vi "voltageScan.vi"(8 "error in (no error)":errorcluster, 11 "VISA Refnum in":refnum<visa-resource-name>) -> (0 "error out":errorcluster, 2 "stringVoltage":string, 3 "numberVoltage":dbl)   [LabVIEW 2018]
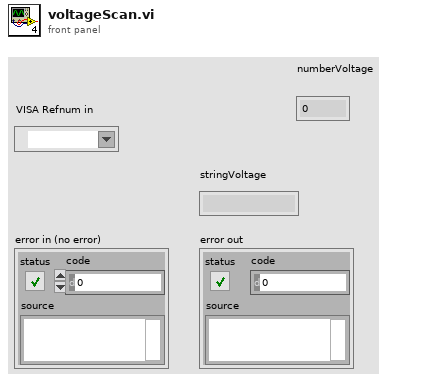
[diagram p1: front panel]
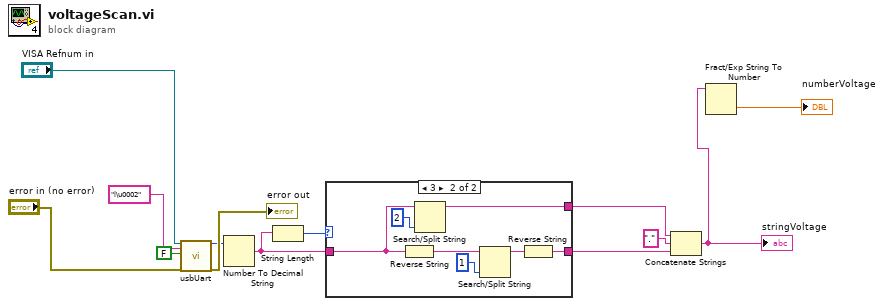
[diagram p0: block diagram]
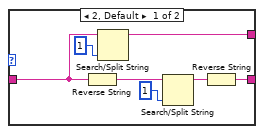
[diagram p2: hidden frame]
diagram:
  n1 = call "usbUart.vi"("VISA resource name"="VISA Refnum in", "write buffer"="l\u0002", "sdFeature"=FALSE, "error in (no error)"="error in (no error)") -> ("number[0]"=w11:u32, "error out"=→"error out":errorcluster)  [unwired: 14 out]
  n2 = Number To Decimal String(number=w11) -> (decimal integer string=w7:string)  [unwired: 1 in]
  n3 = String Length(string=w7) -> (length=w8:i32)
  n4 = case shown="3" w8 {
    tunnel: w7 -> [w14 w21]
    tunnel: [w16 w23] -> w6
    tunnel: [w15 w22] -> w5
    frame 2, Default {
      n5 = Reverse String(1:w14) -> (0:w19:string)
      n6 = Search/Split String(string=w14, offset (0)=1) -> (substring before match=w16:string)  [unwired: 1 in, 2 out]
      n7 = Search/Split String(string=w19, offset (0)=1) -> (substring before match=w20:string)  [unwired: 1 in, 2 out]
      n8 = Reverse String(1:w20) -> (0:w15:string)
    }
    frame 3 {
      n9 = Reverse String(1:w21) -> (0:w26:string)
      n10 = Search/Split String(string=w21, offset (0)=2) -> (substring before match=w23:string)  [unwired: 1 in, 2 out]
      n11 = Search/Split String(string=w26, offset (0)=1) -> (substring before match=w27:string)  [unwired: 1 in, 2 out]
      n12 = Reverse String(1:w27) -> (0:w22:string)
    }
  }
  n13 = Concatenate Strings(w6, "." ("string"), w5) -> (w3:string)
  "stringVoltage" <- w3
  n14 = Fract/Exp String To Number(string=w3) -> (number=→"numberVoltage":dbl)  [unwired: 3 in, 1 out]
